vi "Read Command States Queue.vi"(8 "error in (no error)":errorcluster, 11 "Command Actor in":refnum<class "Command Actor.lvclass">) -> (0 "error out":errorcluster, 2 "Actor Framework:Message Enqueuer":refnum<class "Message Enqueuer.lvclass">, 3 "Command Actor out":refnum<class "Command Actor.lvclass">)   [LabVIEW 2013, in "Command Actor.lvlib" / "Command Actor.lvclass"]
uses:
  Command Actor.lvclass
  <vilib>/ActorFramework/Message Enqueuer/Message Enqueuer.lvclass
  Command Actor.lvclass/Command Actor.ctl
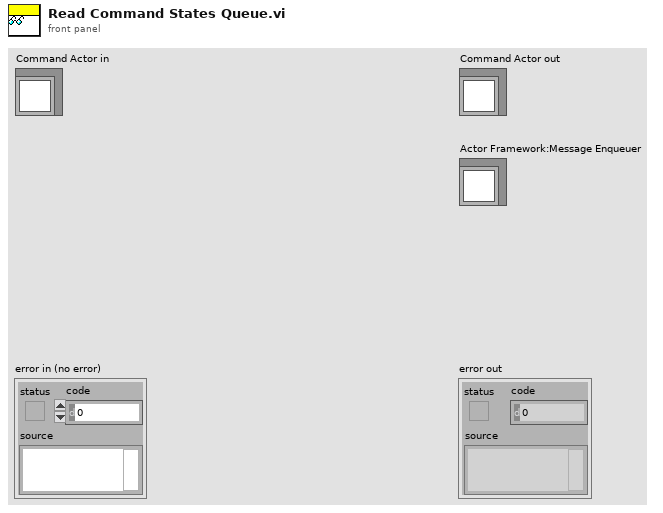
[diagram p1: front panel]
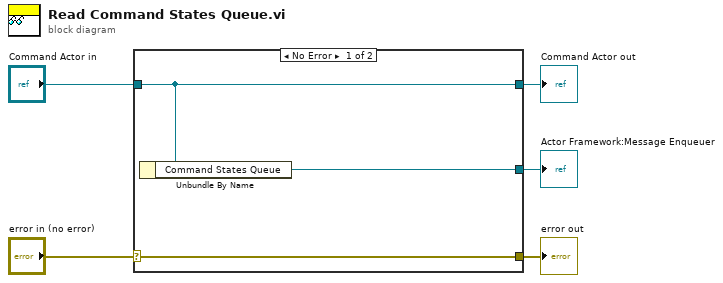
[diagram p0: block diagram]
diagram:
  n1 = case shown="No Error" "error in (no error)" {
    selector: "error in (no error)" -> [w8 w9]
    tunnel: [w8 w9] -> w4
    tunnel: [w7 w10] -> w2
    tunnel: "Command Actor in" -> [w7 w10]
    tunnel: [w6 _] -> w1
    frame No Error {
      n2 = Unbundle By Name(w7) -> ("Command States Queue"=w6:refnum<class "Message Enqueuer.lvclass">)
    }
    frame Error {
    }
  }
  "error out" <- w4
  "Command Actor out" <- w2
  "Actor Framework:Message Enqueuer" <- w1
